vi "Insight_R_Reverse_Index.vi"(8 "error in (no error)":errorcluster, 11 "telnet connection":T1) -> (0 "error out":errorcluster, 1 "response data":string, 2 "Reverse Index":u32, 3 "telnet  connection out":T1)   [LabVIEW 2011]
doc: "Insight Photonic Solutions\n\nThis VI reads the index at which the laser reverses sweep direction, when running in Bidirectional Sweeping mode. This index is the first point of the reversed sweep\n\nver3.2 - original release, but using parser to accept responses from Atlas 3.1 and earlier or Atlas 3.2 and later."
uses:
  Telnet Session.ctl
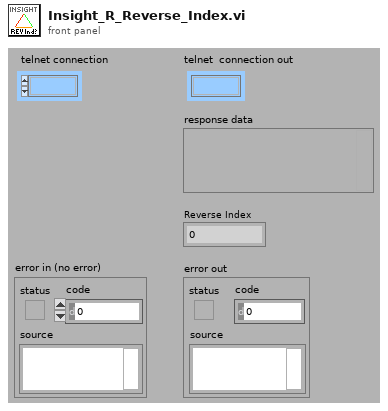
[diagram p1: front panel]
types:
  T1 = typedef "Telnet Session.ctl" = refnum<k1>
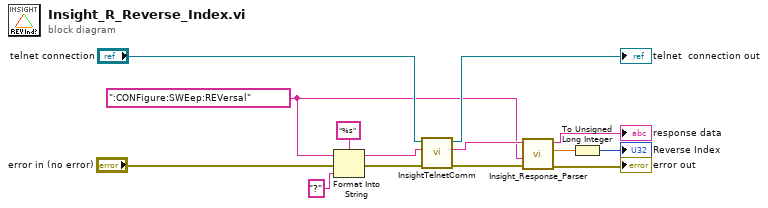
[diagram p0: block diagram]
diagram:
  w2 = ":CONFigure:SWEep:REVersal" ("String")
  n1 = Format Into String(format string="%s", initial string=w2, error in="error in (no error)", "?" ("input 1")) -> (resulting string=w8:string, error out=w11:errorcluster)
  n2 = call "InsightTelnetComm.vi"("error in"=w11, "write buffer (\"\")"=w8, "telnet connection"="telnet connection") -> ("error out"=w3:errorcluster, "response data"=w7:string, "telnet  connection out"=→"telnet  connection out":T1)  [unwired: 4 in]
  n3 = call "Insight_Response_Parser.vi"("error in (no error)"=w3, "Command String"=w2, "Laser Response In"=w7) -> ("error out"=→"error out":errorcluster, "Value"=w5:dbl, "Laser Response Out"=→"response data":string)  [unwired: 6 in]
  n4 = To Unsigned Long Integer(number=w5) -> (unsigned 32bit integer=→"Reverse Index":u32)
